vi "Synchronize 3D.vi"(8 "error in (no error)":errorcluster, 11 "Base in":refnum<class "ODESimulator_LinearConveyor.lvclass">) -> (0 "error out":errorcluster, 3 "Base out":refnum<class "ODESimulator_LinearConveyor.lvclass">)   [LabVIEW 2017, in "NI_Robotics_Simulator.lvlib" / "ODESimulator_LinearConveyor.lvclass"]
uses:
  <vilib>/robotics/Simulator/Robot Factory/Conveyor/Linear/ODESimulator_LinearConveyor.lvclass
  <vilib>/robotics/Simulator/Robot Factory/Conveyor/Linear/ODESimulator_LinearConveyor.lvclass/ODESimulator_LinearConveyor.ctl
  <vilib>/robotics/Simulator/Robot Factory/Conveyor/Base/ODESimulator_Base_Conveyor.lvclass
  <vilib>/picture/3D Picture Control/NI_3D Picture Control.lvlib
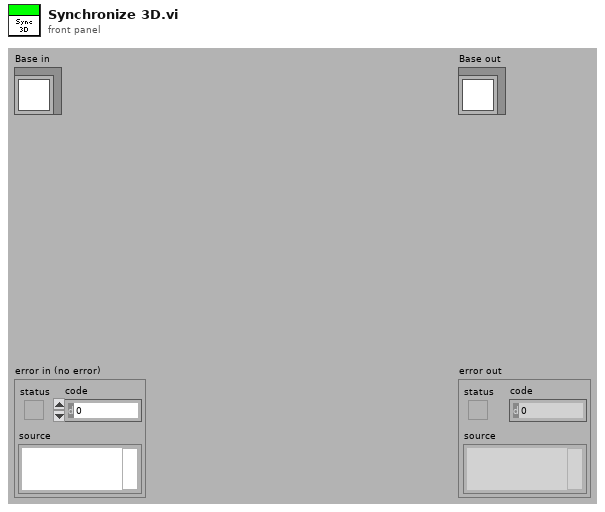
[diagram p1: front panel]
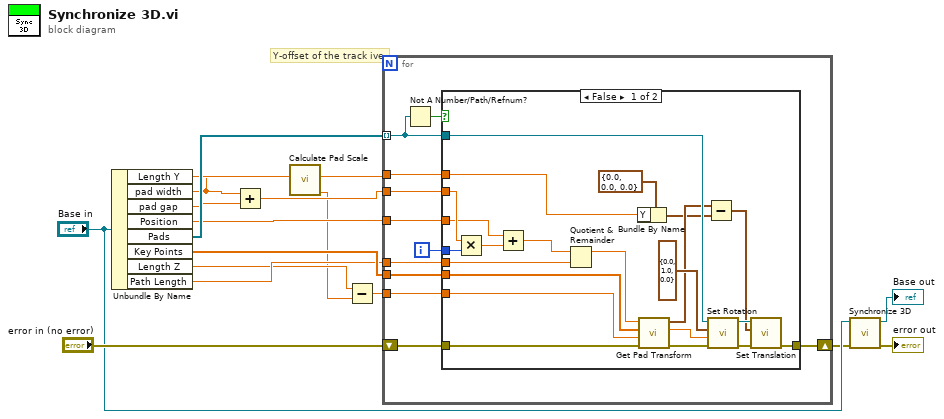
[diagram p0: block diagram]
diagram:
  # "Y-offset of the track ive"
  n1 = Unbundle By Name("Base in") -> ("Length Y"=w4:sgl, "pad width"=w2:dbl, "pad gap"=w13:dbl, "Position"=w14:dbl, "Pads"=w15:refnum<vi>[], "Key Points"=w11:dbl[], "Length Z"=w6:sgl, "Path Length"=w7:dbl)
  n2 = Add(x=w2, y=w13) -> (x+y=w12:dbl)
  n3 = call <vilib>:"Calculate Pad Scale.vi"("Pad width"=w2, "Length Y"=w4) -> ("Z Offset"=w1:sgl, "Y Translation"=w3:sgl)  [unwired: 6 in, 2 out]
  n4 = Subtract(x=w6, y=w1) -> (x-y=w5:sgl)
  n5 = for {
    tunnel: w15 -> [w22] mode=indexing
    tunnel: w14 -> [w26]
    tunnel: w12 -> [w27]
    tunnel: w11 -> [w25]
    shift-right: [w24] -> w8
    shift-left: "error in (no error)" -> [w23]
    tunnel: w7 -> [w20]
    tunnel: w5 -> [w19]
    tunnel: w3 -> [w18]
    i -> [w28]
    n6 = Not A Number/Path/Refnum?(number/path/refnum=w22) -> (NaN/Path/Refnum?=w21:bool)
    n7 = case shown="False" w21 {
      tunnel: w28 -> [w50 _]
      tunnel: w27 -> [w49 _]
      tunnel: w26 -> [w48 _]
      tunnel: w25 -> [w46 _]
      tunnel: [w42 w51] -> w24
      tunnel: w23 -> [w39 w51]
      tunnel: w22 -> [w38 _]
      tunnel: w20 -> [w36 _]
      tunnel: w19 -> [w30 _]
      tunnel: w18 -> [w29 _]
      frame False {
        n8 = Multiply(x=w49, y=w50) -> (x*y=w47:dbl)
        n9 = Add(x=w48, y=w47) -> (x+y=w37:dbl)
        n10 = Quotient & Remainder(x=w37, y=w36) -> (x-y*floor(x/y)=w35:dbl)  [unwired: 1 out]
        n11 = Bundle By Name(cluster=cluster{"X":sgl, "Y":sgl, "Z":sgl} {"X"=0.0, "Y"=0.0, "Z"=0.0} ("x"), "Y"=w29) -> (w32:cluster{"X":sgl, "Y":sgl, "Z":sgl})
        n12 = call <vilib>:"Get Pad Transform.vi"("error in (no error)"=w39, "Length Z"=w30, "Key Points"=w46, "position on path"=w35) -> ("error out"=w40:errorcluster, "angle"=w41:dbl, "translation"=w33:cluster{"X":sgl, "Y":sgl, "Z":sgl})  [unwired: 5 in]
        n13 = Subtract(x=w33, y=w32) -> (x-y=w31:cluster{"X":sgl, "Y":sgl, "Z":sgl})
        n14 = call <vilib>:"Set Rotation.vi"("error in (no error)"=w40, "Angle"=w41, "Axis"=cluster{"X":sgl, "Y":sgl, "Z":sgl} {"X"=0.0, "Y"=1.0, "Z"=0.0}, "Scene Object"=w38) -> ("error out"=w45:errorcluster, "Rotated Scene Object"=w44:refnum<vi>)  [unwired: 6 in]
        n15 = call <vilib>:"Set Translation.vi"("error in (no error)"=w45, "Translation"=w31, "Scene Object"=w44) -> ("error out"=w42:errorcluster)  [unwired: 7 in, 1 out]
      }
      frame True {
      }
    }
  }
  n16 = call-parent "Synchronize 3D.vi"("error in (no error)"=w8, "Base in"="Base in") -> ("error out"=→"error out":errorcluster, "Base out"=→"Base out":refnum<class "ODESimulator_LinearConveyor.lvclass">)  [unwired: 8 in]
